vi "ASCII HEX string TO SYMBOLS string.vi"(8 "error in":errorcluster, 9 "ASCII HEX String":string) -> (0 "error out":errorcluster, 1 "SYMBOLS String":string)   [LabVIEW 2017, in "LV_Unicorn.lvlib"]
uses:
  LV_Unicorn.lvlib
  <vilib>/addons/Tools/Unicode/UTF8 Tools.lvlib
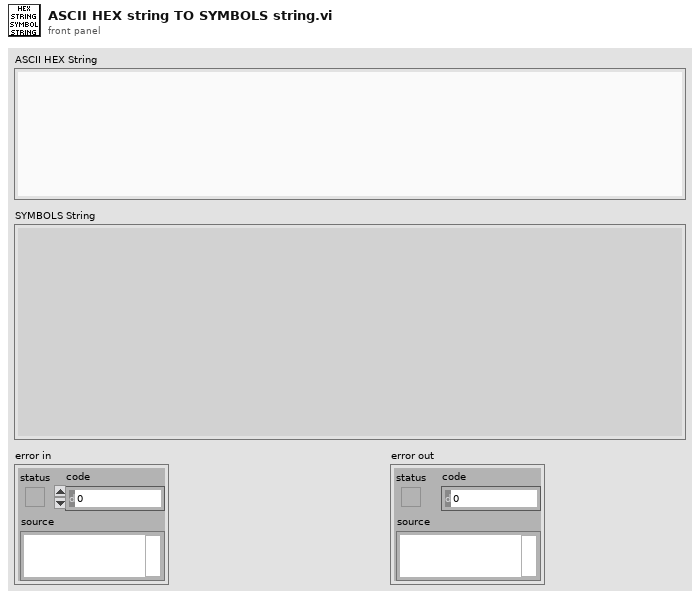
[diagram p1: front panel]
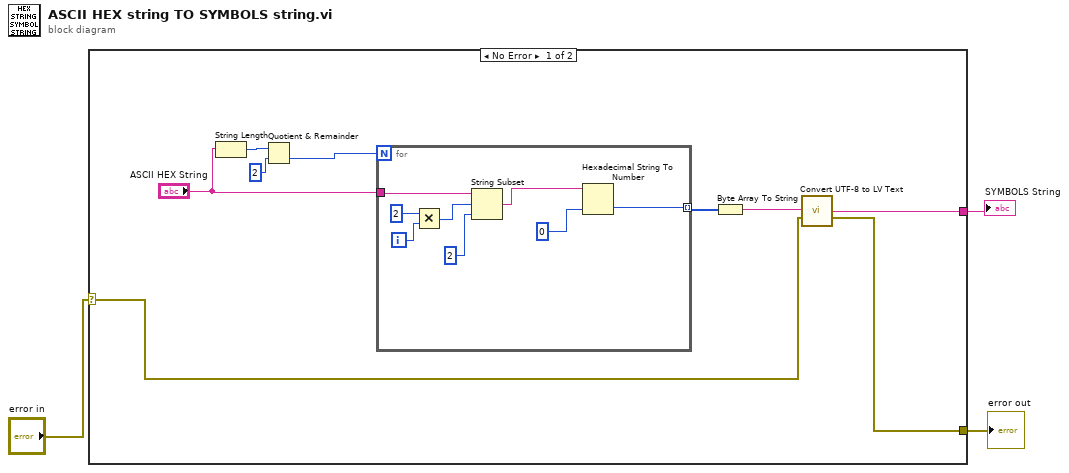
[diagram p0: block diagram]
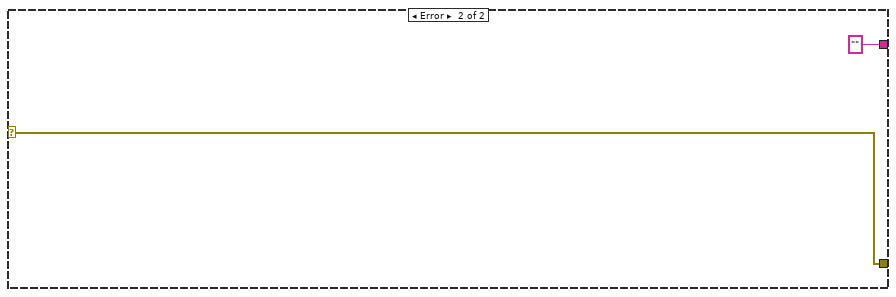
[diagram p2: hidden frame]
diagram:
  n1 = case shown="No Error" "error in" {
    selector: "error in" -> [w4 w21]
    tunnel: [w8 "" ("LV Text")] -> w3
    tunnel: [w5 w21] -> w2
    frame No Error {
      n2 = String Length(string="ASCII HEX String") -> (length=w11:i32)
      n3 = Quotient & Remainder(x=w11, y=2) -> (floor(x/y)=w9:i32)  [unwired: 1 out]
      n4 = for {
        N: w9 -> [_]
        tunnel: "ASCII HEX String" -> [w20]
        tunnel: [w15] -> w7 mode=indexing
        i -> [w14]
        n5 = Multiply(x=2, y=w14) -> (x*y=w18:i32)
        n6 = String Subset(string=w20, offset (0)=w18, length (rest)=2 ("length (rest)")) -> (substring=w16:string)
        n7 = Hexadecimal String To Number(string=w16, default (0uL)=u8 0 ("default (0 U32)")) -> (number=w15:u8)  [unwired: 1 in, 1 out]
      }
      n8 = Byte Array To String(unsigned byte array=w7) -> (string=w6:string)
      n9 = call <vilib>:"Convert UTF-8 to LV Text.vi"("UTF-8 Text"=w6, "error in"=w4) -> ("LV Text"=w8:string, "error out"=w5:errorcluster)  [unwired: 12 in]
    }
    frame Error {
    }
  }
  "SYMBOLS String" <- w3
  "error out" <- w2
